vi "Main.vi"() -> ()   [LabVIEW 2014, in "TestFramework.lvlib"]
uses:
  TestFramework.lvlib
  FrontPanel/TypeDefs/clFrontPanelControlRefs.ctl
  WfrmGenerator/WfrmModule/WfrmModule.lvlib
  FGenModule/FGenModule.lvlib
  Bus/NISTBus.lvclass
  <userlib>/NIST/NISTErrorLib/NISTErrorLib.lvlib
  <vilib>/Utility/error.llb/Error Cluster From Error Code.vi
  <vilib>/ErrorRing/Error Ring.xnode
  FGenModule/PublicAPI/Arguments/Broadcasts/clErrorRpt.ctl
  WfrmGenerator/WfrmModule/PublicAPI/Arguments/Broadcasts/clErrorRpt.ctl
  WfrmGenerator/WfrmPlugins/EventPluginBaseClass/TypeDefs/dblEvtSignalArray.ctl
  WfrmGenerator/WfrmPlugins/EventPluginBaseClass/BaseWfrmPlugin.lvclass
  FGenPlugins/MyPluginBaseClass/TypeDef/PluginParams.ctl
  FGenPlugins/MyPluginBaseClass/NISTFGenPluginsBase.lvclass
  WfrmGenerator/WfrmPlugins/EventPluginBaseClass/TypeDefs/clEvtConfig.ctl
  WfrmGenerator/WfrmModule/PublicAPI/Arguments/Requests/dblEvtParams.ctl
  FGenPlugins/MyPluginBaseClass/TypeDef/CreateArbWfrmParams.ctl
  FGenPlugins/MyPluginBaseClass/TypeDef/ConfigArbWfrmParams.ctl
  FGenPlugins/MyPluginBaseClass/TypeDef/TriggerParams.ctl
panel:
  in  "btnSetTrigger":bool caption="btnLoadPlugin"
  in  "TriggerParams":T1={"eTrigger"=0, "eEdge"=10280, "sSource"=""} {"eEdge" items=["Rising"=10280, "Falling"=10171]; "eTrigger" items=["None", "Digital", "Analog"]}
  in  "EndTime":dbl=1.0
  in  "StartTime":dbl
  in  "btnClearArbWfrm":bool
  in  "ClrArbWfrmParams":cluster{"iIndex":i32}
  in  "btnInitialize":bool
  in  "btnReset":bool
  in  "btnSetOutputEnable":bool caption="btnLoadPlugin"
  in  "OutputEnableParams":cluster{"sName":string, "bEnabled":bool}
  in  "ConfigArbWfrmParams":T2={"sName"="1", "dGain"=2.0, "sWfrmHandle"="ARB1", "dOffset"=-1.0, "dSampleRate"=10000.0}
  in  "btnConfigWaveform":bool caption="btnLoadPlugin"
  in  "CreateArbWfrmParams":T3={"sName"="1", "iSize"=10000, "dData"=[], "sWfrmHandle"="ARB1"}
  in  "btnSendWaveform":bool caption="btnLoadPlugin"
  out "dblEventSignalArray":T4
  in  "dblEvtParams":T5=[[70.0, 70.0, 70.0, 70.0, 20.0, 20.0, 20.0, 20.0], [50.0, 60.0, 60.0, 60.0, 60.0, 60.0, 60.0, 60.0], [0.0, 0.0, 0.0, 0.0, 0.0, 0.0, 0.0, 0.0], [0.0, 0.0, 0.0, 0.0, 0.0, 0.0, 0.0, 0.0], [0.0, 0.0, 0.0, 0.0, 0.0, 0.0, 0.0, 0.0], [0.0, 0.0, 0.0, 0.0, 0.0, 0.0, 0.0, 0.0], [0.0, 0.0, 0.0, 0.0, 0.0, 0.0, 0.0, 0.0], [0.0, 0.0, 0.0, 0.0, 0.0, 0.0, 0.0, 0.0], [0.0, 0.0, 0.0, 0.0, 0.0, 0.0, 0.0, 0.0], [0.0, 0.0, 0.0, 0.0, 0.0, 0.0, 0.0, 0.0], [0.0, 0.0, 0.0, 0.0, 0.0, 0.0, 0.0, 0.0], [0.0, 0.0, 0.0, 0.0, 0.0, 0.0, 0.0, 0.0], [0.0, 0.0, 0.0, 0.0, 0.0, 0.0, 0.0, 0.0]]
  in  "clEvtConfig":T6={"T0(UTC)"=0.0, "F0"=60.0, "Fs"=60, "FSamp"=10000}
  in  "btnCreateWaveform":bool caption="btnLoadPlugin"
  in  "btnLoadWaveformPlugin":bool caption="btnLoadPlugin"
  in  "btnLoadPlugin":bool
  in  "Path to INI Waveform Plugin":path=path "../../EventPlugins/C37EvtPlugin/C37EvtPlugin.ini"
  in  "PluginParams":T7={"Path to Plugin INI"=path "../../MyPlugins/NiPxi6733/NiPxi6733.ini"}
  in  "btnRemoveBus":bool
  in  "btnSingleRun":bool
  out "Number of Buses":u8
  in  "Bus Number":u8(ring)
  in  "btnExit":bool
  in  "btnAddBus":bool
  # "Xm\nFin\nPs\nFh\nPh\nKh\nFa\nKa\nFx\nKx\nRf\nKaS\nKxS"
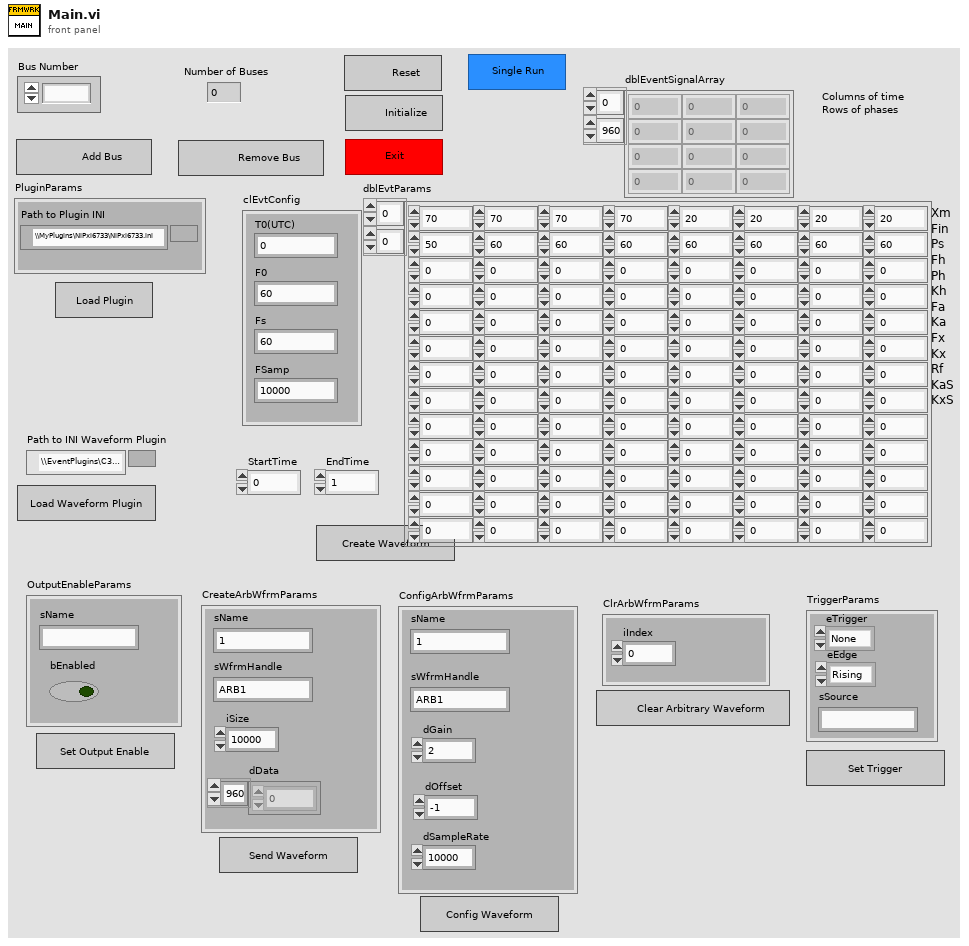
[diagram p1: front panel]
types:
  T1 = typedef "FGenPlugins.lvlib/NISTFGenPluginsBase.lvclass/TriggerParams.ctl" = cluster{"eTrigger":u16, "eEdge":u16, "sSource":string}
  T2 = typedef "FGenPlugins.lvlib/NISTFGenPluginsBase.lvclass/ConfigArbWfrmParams.ctl" = cluster{"sName":string, "dGain":dbl, "sWfrmHandle":string, "dOffset":dbl, "dSampleRate":dbl}
  T3 = typedef "FGenPlugins.lvlib/NISTFGenPluginsBase.lvclass/CreateArbWfrmParams.ctl" = cluster{"sName":string, "iSize":i32, "dData":dbl[], "sWfrmHandle":string}
  T4 = typedef "WfrmPlugins.lvlib/BaseWfrmPlugin.lvclass/dblEvtSignalArray.ctl" = dbl[][]
  T5 = typedef "WfrmModule.lvlib/dblEvtParams.ctl" = dbl[][]
  T6 = typedef "WfrmPlugins.lvlib/BaseWfrmPlugin.lvclass/clEvtConfig.ctl" = cluster{"T0(UTC)":dbl, "F0":dbl, "Fs":i32, "FSamp":u32}
  T7 = typedef "FGenPlugins.lvlib/NISTFGenPluginsBase.lvclass/PluginParams.ctl" = cluster{"Path to Plugin INI":path}
  T8 = typedef "TestFramework.lvlib/clFrontPanelControlRefs.ctl" = cluster{"BusNumberRef":refnum<vi>, "NumberOfBusesRef":refnum<vi>, "FGenPluginParamsRef":refnum<vi>, "WfrmINIFilePath":refnum<vi>, "EventSignalArrayRef":refnum<vi>, "CreateArbWfrmRef":refnum<vi>, "clEvtConFigRef":refnum<vi>, "dblEvtParamsRef":refnum<vi>, "clOutputEnableParamsRef":refnum<vi>, "ConfigArbWfrmRef":refnum<vi>, "ClArbWfrmParamsRef":refnum<vi>, "dStartTimeRef":refnum<vi>, "dEndTimeRef":refnum<vi>, "TriggerParamsRef":refnum<vi>}
  T9 = typedef "FGenModule.lvlib/clBroadcastEvents.ctl" = cluster{"DidInit":refnum<user-event>, "StatusUpdate":refnum<user-event>, "ErrorReport":refnum<user-event>, "DidStop":refnum<user-event>, "PathToINI":refnum<user-event>, "ChannelName":refnum<user-event>}
  T10 = typedef "WfrmModule.lvlib/clBroadcastEvents.ctl" = cluster{"DidInit":refnum<user-event>, "StatusUpdate":refnum<user-event>, "ErrorReport":refnum<user-event>, "DidStop":refnum<user-event>, "ReadEvtConfig":refnum<user-event>, "ReadTimeArray":refnum<user-event>, "ReadEvtParams":refnum<user-event>, "GetEvtReportArray":refnum<user-event>, "ReadPathToPlugin":refnum<user-event>, "GetEvtSignal":refnum<user-event>, "SendArbWfrm":refnum<user-event>}
  T11 = typedef "TestFramework.lvlib/clRequestEvents.ctl" = cluster{"StopRequest":refnum<user-event>}
  T12 = typedef "FGenModule.lvlib/clErrorRpt.ctl" = cluster{"error":errorcluster, "AdditionalInfo":string}
  T13 = typedef "WfrmModule.lvlib/clErrorRpt.ctl" = cluster{"error":errorcluster, "AdditionalInfo":string}
  T14 = typedef "TestFramework.lvlib/QueRef.ctl" = refnum<queue>
  T15 = typedef "TestFramework.lvlib/clFrameworkData.ctl" = cluster{"NISTBusClassInstances":refnum<class "NISTBus.lvclass">[], "NISTFGenINIFilePaths":path[], "NISTWfrmINIFilePaths":path[]}
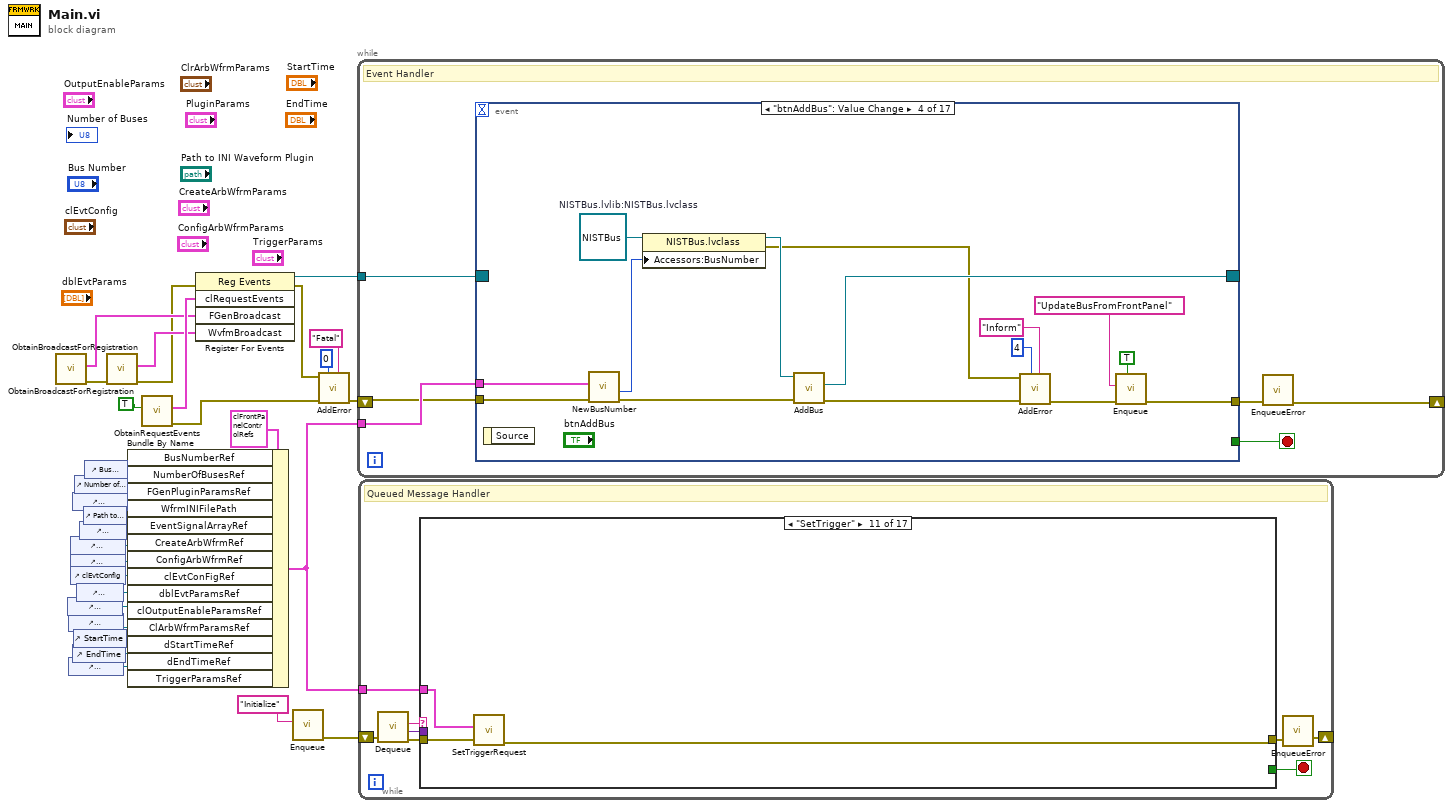
[diagram p0: block diagram]
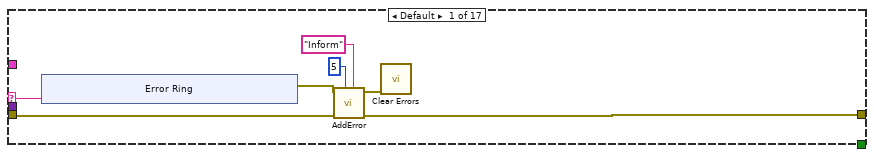
[diagram p2: hidden frame]
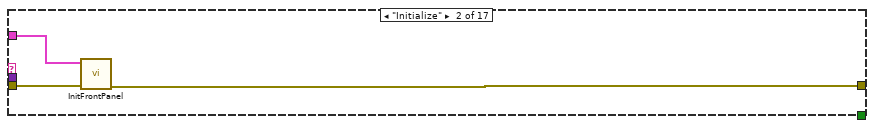
[diagram p3: hidden frame]
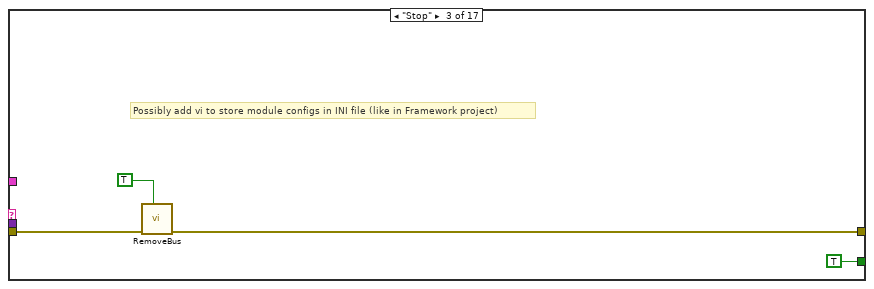
[diagram p4: hidden frame]
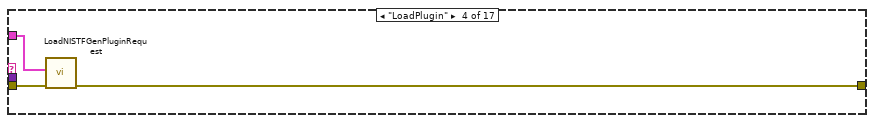
[diagram p5: hidden frame]
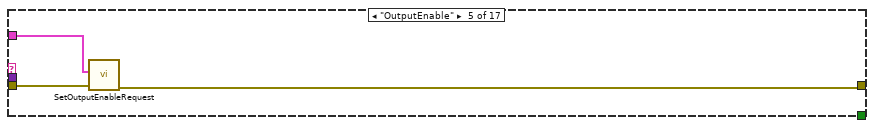
[diagram p6: hidden frame]
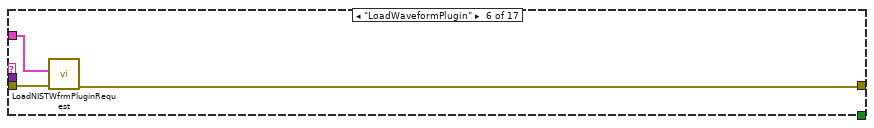
[diagram p7: hidden frame]
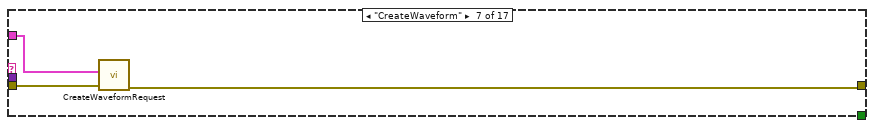
[diagram p8: hidden frame]
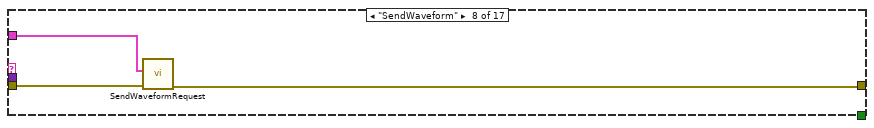
[diagram p9: hidden frame]
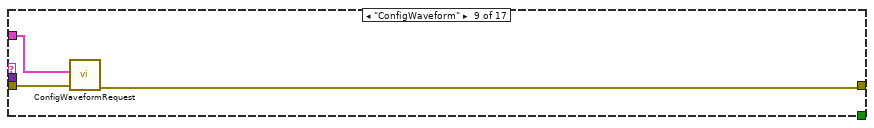
[diagram p10: hidden frame]
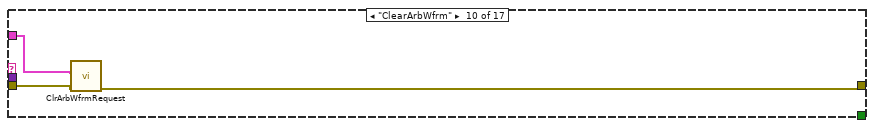
[diagram p11: hidden frame]
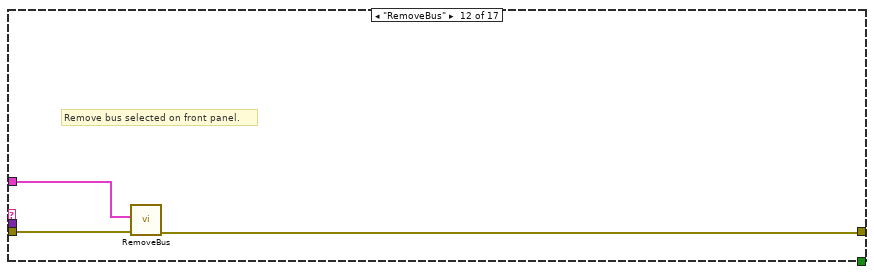
[diagram p12: hidden frame]
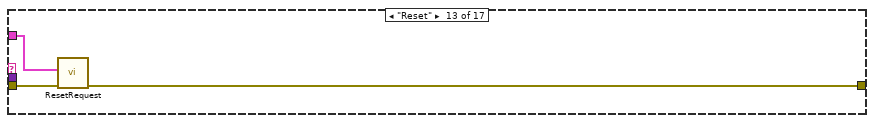
[diagram p13: hidden frame]
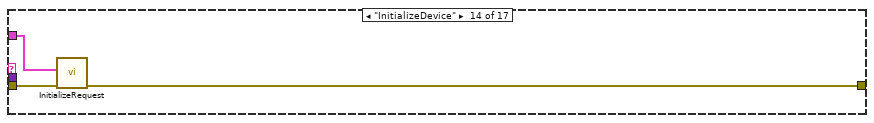
[diagram p14: hidden frame]
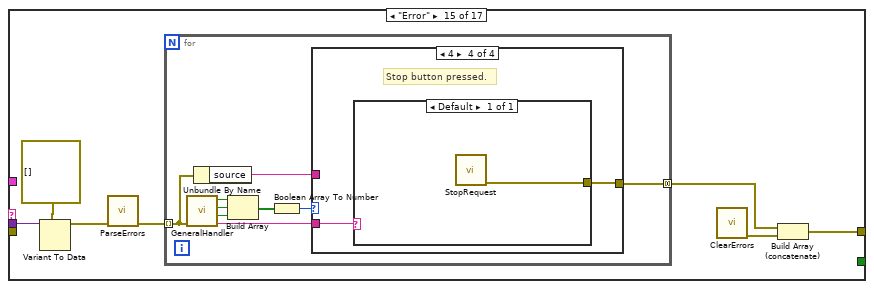
[diagram p15: hidden frame]
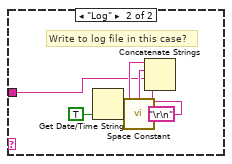
[diagram p18: hidden frame]
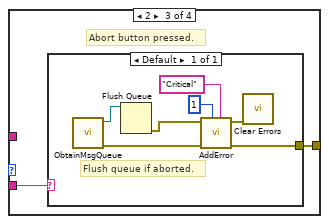
[diagram p19: hidden frame]
diagram:
  n1 = call "ObtainBroadcastForRegistration.vi"() -> ("error out"=w25:errorcluster, "FGenBroadcast"=w23:T9)  [unwired: 10 in]
  n2 = control-ref of="OutputEnableParams"() -> (w6:refnum<vi>)
  n3 = control-ref of="ClrArbWfrmParams"() -> (w4:refnum<vi>)
  n4 = control-ref of="TriggerParams"() -> (w1:refnum<vi>)
  n5 = control-ref of="CreateArbWfrmParams"() -> (w9:refnum<vi>)
  n6 = control-ref of="ConfigArbWfrmParams"() -> (w5:refnum<vi>)
  n7 = control-ref of="clEvtConfig"() -> (w8:refnum<vi>)
  n8 = control-ref of="PluginParams"() -> (w12:refnum<vi>)
  n9 = control-ref of="EndTime"() -> (w2:refnum<vi>)
  n10 = control-ref of="StartTime"() -> (w3:refnum<vi>)
  n11 = control-ref of="Number of Buses"() -> (w28:refnum<vi>)
  n12 = control-ref of="dblEvtParams"() -> (w7:refnum<vi>)
  n13 = control-ref of="dblEventSignalArray"() -> (w10:refnum<vi>)
  n14 = control-ref of="Path to INI Waveform Plugin"() -> (w11:refnum<vi>)
  n15 = control-ref of="Bus Number"() -> (w29:refnum<vi>)
  n16 = call "ObtainBroadcastForRegistration.vi"("error in (no error)"=w25) -> ("error out"=w22:errorcluster, "WvfmBroadcast"=w24:T10)  [unwired: 9 in]
  n17 = Bundle By Name(cluster=T8 {"BusNumberRef"=refnum, "NumberOfBusesRef"=refnum, "FGenPluginParamsRef"=refnum, "WfrmINIFilePath"=refnum, "EventSignalArrayRef"=refnum, "CreateArbWfrmRef"=refnum, "clEvtConFigRef"=refnum, "dblEvtParamsRef"=refnum, "clOutputEnableParamsRef"=refnum, "ConfigArbWfrmRef"=refnum, "ClArbWfrmParamsRef"=refnum, "dStartTimeRef"=refnum, "dEndTimeRef"=refnum, "TriggerParamsRef"=refnum} ("clFrontPanelControlRefs"), "BusNumberRef"=w29, "NumberOfBusesRef"=w28, "FGenPluginParamsRef"=w12, "WfrmINIFilePath"=w11, "EventSignalArrayRef"=w10, "CreateArbWfrmRef"=w9, "ConfigArbWfrmRef"=w5, "clEvtConFigRef"=w8, "dblEvtParamsRef"=w7, "clOutputEnableParamsRef"=w6, "ClArbWfrmParamsRef"=w4, "dStartTimeRef"=w3, "dEndTimeRef"=w2, "TriggerParamsRef"=w1) -> (w13:T8)
  n18 = call "ObtainRequestEvents.vi"("CreateNew (F)"=TRUE) -> ("ErrorArray Out"=w16:errorcluster[], "clRequestEvents"=w26:T11)  [unwired: 9 in]
  n19 = register-events(error in=w22, w26, w23, w24) -> (reference out=w21:refnum<event-registration>, error out=w17:errorcluster)  [unwired: 1 in]
  n20 = call "Enqueue.vi"("Msg"="Initialize") -> ("ErrorArray Out"=w14:errorcluster[])  [unwired: 10 in]
  n21 = call <userlib>:"AddError.vi"("Severity"="Fatal" ("String"), "Priority"=u8 0, "ErrorArray"=w16, "error in (no error)"=w17) -> ("ErrorArray"=w18:errorcluster[])  [unwired: 6 in, 1 out]
  n22 = while {
    tunnel: w21 -> [w35]
    tunnel: w13 -> [w34]
    shift-right: [w31] -> _
    shift-left: w18 -> [w33]
    stop <- w36 stop-if-true
    # "Event Handler"
    n23 = event shown="[3] \"btnAddBus\": Value Change" {
      selector: w35 -> [_ _ _ _ _ _ _ _ _ _ _ _ _ _ _ _ _]
      dyn-events: [_ _ _ w70 _ _ _ _ _ _ _ _ _ _ _ _ _] -> _
      timeout: _ -> [_ _ _ _ _ _ _ _ _ _ _ _ _ _ _ _ _]
      tunnel: [TRUE _ _ _ _ _ _ _ _ _ _ _ _ _ _ _ _] -> w36
      tunnel: w34 -> [_ _ _ w76 _ _ _ _ _ _ _ _ _ _ _ _ _]
      tunnel: w33 -> [w42 w45 w55 w73 w80 w83 w86 w89 w92 w95 w98 w101 w103 w106 w109 w113 w118]
      tunnel: [w39 w44 w54 w64 w79 w82 w85 w88 w91 w94 w97 w100 w102 w105 w108 w112 w117] -> w32
      event "btnExit": Value Change {
        n24 = event-data() -> ()  [unwired: 1 in, 1 out]
        n25 = call "RemoveBus.vi"("Remove All? (F)"=TRUE, "ErrorArray In"=w42) -> ("ErrorArray Out"=w40:errorcluster[])  [unwired: 9 in]
        n26 = call "Enqueue.vi"("Priority (f)"=TRUE, "ErrorArray In"=w40, "Msg"="Stop") -> ("ErrorArray Out"=w39:errorcluster[])  [unwired: 8 in]
      }
      event User Event {
        n27 = event-data() -> ("Data"=w46:variant)  [unwired: 1 in]
        n28 = Variant To Data(type=T12 {"error"={"status"=FALSE, "code"=0, "source"=""}, "AdditionalInfo"=""} ("Cluster"), Variant=w46) -> (data=w52:T12)  [unwired: 1 in, 1 out]
        n29 = Unbundle By Name(w52) -> ("error"=w48:errorcluster)
        n30 = call <userlib>:"AddError.vi"("Severity"="UserOption" ("String"), "Priority"=u8 2, "ErrorArray"=w45, "error in (no error)"=w48) -> ("ErrorArray"=w44:errorcluster[], "error out"=w49:errorcluster)  [unwired: 6 in]
        n31 = call <vilib>:"Clear Errors.vi"("error in (no error)"=w49) -> ()  [unwired: 5 in, 2 out]
      }
      event User Event {
        n32 = event-data() -> ("Data"=w61:variant)  [unwired: 1 in]
        n33 = Variant To Data(type=T13 {"error"={"status"=FALSE, "code"=0, "source"=""}, "AdditionalInfo"=""} ("Cluster"), Variant=w61) -> (data=w59:T13)  [unwired: 1 in, 1 out]
        n34 = Unbundle By Name(w59) -> ("error"=w53:errorcluster)
        n35 = call <userlib>:"AddError.vi"("Severity"="UserOption" ("String"), "Priority"=u8 2, "ErrorArray"=w55, "error in (no error)"=w53) -> ("ErrorArray"=w54:errorcluster[], "error out"=w56:errorcluster)  [unwired: 6 in]
        n36 = call <vilib>:"Clear Errors.vi"("error in (no error)"=w56) -> ()  [unwired: 5 in, 2 out]
      }
      event "btnAddBus": Value Change {
        w75 = refnum<class "NISTBus.lvclass"> refnum  # NISTBus.lvlib:NISTBus.lvclass
        n37 = event-data() -> ()  [unwired: 1 in, 1 out]
        n38 = call "NewBusNumber.vi"("ErrorArray In"=w73, "clFrontPanelControlRefs In"=w76) -> ("ErrorArray Out"=w71:errorcluster[], "BusNumber"=w74:u8)  [unwired: 7 in, 1 out]
        n39 = property class="NISTBus.lvclass"(reference=w75, "Accessors:BusNumber"=w74) -> (reference out=w72:refnum<class "NISTBus.lvclass">, error out=w67:errorcluster)  [unwired: 1 in]
        n40 = call "AddBus.vi"("ErrorArray In"=w71, "NISTBusClass In"=w72) -> ("ErrorArray Out"=w66:errorcluster[], "EvtReg"=w70:refnum<event-registration>)  [unwired: 7 in, 1 out]
        n41 = call <userlib>:"AddError.vi"("Severity"="Inform" ("String"), "Priority"=u8 4, "ErrorArray"=w66, "error in (no error)"=w67) -> ("ErrorArray"=w65:errorcluster[])  [unwired: 6 in, 1 out]
        n42 = call "Enqueue.vi"("Priority (f)"=TRUE, "ErrorArray In"=w65, "Msg"="UpdateBusFromFrontPanel") -> ("ErrorArray Out"=w64:errorcluster[])  [unwired: 8 in]
      }
      event "btnRemoveBus": Value Change {
        n43 = event-data() -> ()  [unwired: 1 in, 1 out]
        n44 = call "Enqueue.vi"("Priority (f)"=TRUE, "ErrorArray In"=w80, "Msg"="RemoveBus") -> ("ErrorArray Out"=w79:errorcluster[])  [unwired: 8 in]
      }
      event "btnReset": Value Change {
        n45 = event-data() -> ()  [unwired: 1 in, 1 out]
        n46 = call "Enqueue.vi"("ErrorArray In"=w83, "Msg"="Reset") -> ("ErrorArray Out"=w82:errorcluster[])  [unwired: 9 in]
      }
      event "btnInitialize": Value Change {
        n47 = event-data() -> ()  [unwired: 1 in, 1 out]
        n48 = call "Enqueue.vi"("ErrorArray In"=w86, "Msg"="InitializeDevice") -> ("ErrorArray Out"=w85:errorcluster[])  [unwired: 9 in]
      }
      event "btnSingleRun": Value Change {
        n49 = event-data() -> ()  [unwired: 1 in, 1 out]
        n50 = call "Enqueue.vi"("ErrorArray In"=w89, "Msg"="SingleRun") -> ("ErrorArray Out"=w88:errorcluster[])  [unwired: 9 in]
      }
      event "btnLoadPlugin": Value Change {
        n51 = event-data() -> ()  [unwired: 1 in, 1 out]
        n52 = call "Enqueue.vi"("ErrorArray In"=w92, "Msg"="LoadPlugin") -> ("ErrorArray Out"=w91:errorcluster[])  [unwired: 9 in]
      }
      event "btnSetOutputEnable": Value Change {
        n53 = event-data() -> ()  [unwired: 1 in, 1 out]
        n54 = call "Enqueue.vi"("ErrorArray In"=w95, "Msg"="OutputEnable") -> ("ErrorArray Out"=w94:errorcluster[])  [unwired: 9 in]
      }
      event "btnLoadWaveformPlugin": Value Change {
        n55 = event-data() -> ()  [unwired: 1 in, 1 out]
        n56 = call "Enqueue.vi"("ErrorArray In"=w98, "Msg"="LoadWaveformPlugin") -> ("ErrorArray Out"=w97:errorcluster[])  [unwired: 9 in]
      }
      event "btnCreateWaveform": Value Change {
        n57 = event-data() -> ()  [unwired: 1 in, 1 out]
        n58 = call "Enqueue.vi"("ErrorArray In"=w101, "Msg"="CreateWaveform") -> ("ErrorArray Out"=w100:errorcluster[])  [unwired: 9 in]
      }
      event "btnSendWaveform": Value Change {
        n59 = event-data() -> ()  [unwired: 1 in, 1 out]
        n60 = call "Enqueue.vi"("ErrorArray In"=w103, "Msg"="SendWaveform") -> ("ErrorArray Out"=w102:errorcluster[])  [unwired: 9 in]
      }
      event "btnConfigWaveform": Value Change {
        n61 = event-data() -> ()  [unwired: 1 in, 1 out]
        n62 = call "Enqueue.vi"("ErrorArray In"=w106, "Msg"="ConfigWaveform") -> ("ErrorArray Out"=w105:errorcluster[])  [unwired: 9 in]
      }
      event "btnClearArbWfrm": Value Change {
        n63 = event-data() -> ()  [unwired: 1 in, 1 out]
        n64 = call "Enqueue.vi"("ErrorArray In"=w109, "Msg"="ClearArbWfrm") -> ("ErrorArray Out"=w108:errorcluster[])  [unwired: 9 in]
      }
      event "btnSetTrigger": Value Change {
        n65 = event-data() -> ()  [unwired: 1 in, 1 out]
        n66 = call "Enqueue.vi"("ErrorArray In"=w113, "Msg"="SetTrigger") -> ("ErrorArray Out"=w112:errorcluster[])  [unwired: 9 in]
      }
      event User Event {
        n67 = event-data() -> ("Data"=w121:variant)  [unwired: 1 in]
        n68 = Variant To Data(type=T4 [] ("dblEventSignalArray"), Variant=w121) -> (data=→"dblEventSignalArray":T4, error out=w116:errorcluster)  [unwired: 1 in]
        n69 = call <userlib>:"AddError.vi"("Severity"="Inform" ("String"), "Priority"=u8 4, "ErrorArray"=w118, "error in (no error)"=w116) -> ("ErrorArray"=w117:errorcluster[])  [unwired: 6 in, 1 out]
      }
    }
    n70 = call "EnqueueError.vi"("ErrorArray In"=w32) -> ("ErrorArray Out"=w31:errorcluster[])  [unwired: 10 in]
  }
  n71 = while {
    shift-right: [w124] -> _
    shift-left: w14 -> [w128]
    tunnel: w13 -> [w129]
    stop <- w122 stop-if-true
    # "Queued Message Handler"
    n72 = call "Dequeue.vi"("ErrorArray In"=w128) -> ("ErrorArray Out"=w125:errorcluster[], "Data"=w126:variant, "Msg"=w127:string)  [unwired: 8 in]
    n73 = case shown="\"SetTrigger\"" w127 {
      selector: w127 -> [w130 _ _ _ _ _ _ _ _ _ _ _ _ _ _ _ _]
      tunnel: w129 -> [_ w146 _ w151 w154 w157 w160 w163 w166 w170 w173 w176 w180 w181 _ _ _]
      tunnel: w126 -> [_ _ _ _ _ _ _ _ _ _ _ _ _ _ w190 _ _]
      tunnel: w125 -> [w132 w145 w150 w153 w156 w159 w162 w165 w168 w169 w174 w177 w179 w182 _ w219 _]
      tunnel: [w131 w144 w149 w152 w155 w158 w161 w164 w167 w171 w172 w175 w178 w183 w185 w219 w220] -> w123
      tunnel: [_ _ TRUE _ _ _ _ _ _ _ _ _ _ _ _ _ _] -> w122
      frame Default {
        n74 = xnode "Error Ring"("parameter 0"=w130) -> ("error out"=w136:errorcluster)
        n75 = call <userlib>:"AddError.vi"("Severity"="Inform" ("String"), "Priority"=u8 5, "ErrorArray"=w132, "error in (no error)"=w136) -> ("ErrorArray"=w131:errorcluster[], "error out"=w133:errorcluster)  [unwired: 6 in]
        n76 = call <vilib>:"Clear Errors.vi"("error in (no error)"=w133) -> ()  [unwired: 5 in, 2 out]
      }
      frame "Initialize" {
        n77 = call "InitFrontPanel.vi"("ErrorArray In"=w145, "clFrontPanelControlRefs"=w146) -> ("ErrorArray Out"=w144:errorcluster[])  [unwired: 9 in]
      }
      frame "Stop" {
        # "Possibly add vi to store module configs in INI file (like in Framework project)"
        n78 = call "RemoveBus.vi"("Remove All? (F)"=TRUE, "ErrorArray In"=w150) -> ("ErrorArray Out"=w149:errorcluster[])  [unwired: 9 in]
      }
      frame "LoadPlugin" {
        n79 = call "LoadNISTFGenPluginRequest.vi"("ErrorArray In"=w153, "clFrontPanelControlRefs"=w151) -> ("ErrorArray Out"=w152:errorcluster[])  [unwired: 9 in]
      }
      frame "OutputEnable" {
        n80 = call "SetOutputEnableRequest.vi"("ErrorArray In"=w156, "clFrontPanelControlRefs"=w154) -> ("ErrorArray Out"=w155:errorcluster[])  [unwired: 9 in]
      }
      frame "LoadWaveformPlugin" {
        n81 = call "LoadNISTWfrmPluginRequest.vi"("ErrorArray In"=w159, "clFrontPanelControlRefs"=w157) -> ("ErrorArray Out"=w158:errorcluster[])  [unwired: 9 in]
      }
      frame "CreateWaveform" {
        n82 = call "CreateWaveformRequest.vi"("ErrorArray In"=w162, "clFrontPanelControlRefs"=w160) -> ("ErrorArray Out"=w161:errorcluster[])  [unwired: 9 in]
      }
      frame "SendWaveform" {
        n83 = call "SendWaveformRequest.vi"("ErrorArray In"=w165, "clFrontPanelControlRefs"=w163) -> ("ErrorArray Out"=w164:errorcluster[])  [unwired: 9 in]
      }
      frame "ConfigWaveform" {
        n84 = call "ConfigWaveformRequest.vi"("ErrorArray In"=w168, "clFrontPanelControlRefs"=w166) -> ("ErrorArray Out"=w167:errorcluster[])  [unwired: 9 in]
      }
      frame "ClearArbWfrm" {
        n85 = call "ClrArbWfrmRequest.vi"("ErrorArray In"=w169, "clFrontPanelControlRefs"=w170) -> ("ErrorArray Out"=w171:errorcluster[])  [unwired: 9 in]
      }
      frame "SetTrigger" {
        n86 = call "SetTriggerRequest.vi"("ErrorArray In"=w174, "clFrontPanelControlRefs"=w173) -> ("ErrorArray Out"=w172:errorcluster[])  [unwired: 9 in]
      }
      frame "RemoveBus" {
        # "Remove bus selected on front panel."
        n87 = call "RemoveBus.vi"("ErrorArray In"=w177, "clFrontPanelControlRefs"=w176) -> ("ErrorArray Out"=w175:errorcluster[])  [unwired: 9 in]
      }
      frame "Reset" {
        n88 = call "ResetRequest.vi"("ErrorArray In"=w179, "clFrontPanelControlRefs"=w180) -> ("ErrorArray Out"=w178:errorcluster[])  [unwired: 9 in]
      }
      frame "InitializeDevice" {
        n89 = call "InitializeRequest.vi"("ErrorArray In"=w182, "clFrontPanelControlRefs"=w181) -> ("ErrorArray Out"=w183:errorcluster[])  [unwired: 9 in]
      }
      frame "Error" {
        n90 = Variant To Data(type=errorcluster[] [], Variant=w190) -> (data=w188:errorcluster[])  [unwired: 1 in, 1 out]
        n91 = call <userlib>:"ParseErrors.vi"("ErrorArray"=w188) -> ("ErrorArray"=w187:errorcluster[])  [unwired: 8 in, 2 out]
        n92 = for {
          tunnel: w187 -> [w199] mode=indexing
          tunnel: [w191] -> w184 mode=concatenating
          n93 = call <userlib>:"GeneralHandler.vi"("error in (no error)"=w199) -> ("Severity"=w192:string, "Stop"=w196:bool, "Abort"=w197:bool, "Continue"=w198:bool)  [unwired: 7 in]
          n94 = Unbundle By Name(w199) -> ("source"=w193:string)
          n95 = Build Array(w198, w197, w196) -> (w194:bool[])
          n96 = Boolean Array To Number(Boolean array=w194) -> (number=w195:u32)
          n97 = case shown="4" w195 {
            tunnel: w193 -> [_ w200 _ _]
            tunnel: w192 -> [_ w201 w208 w217]
            tunnel: [_ _ w207 w216] -> w191
            frame 0, Default {
              # "No dialogue button pressed."
            }
            frame 1 {
              # "Continue button pressed."
              n98 = case shown="Default" w201 {
                tunnel: w200 -> [_ w202]
                frame Default {
                  # "Let the Framework continue."
                }
                frame "Log" {
                  # "Write to log file in this case?"
                  n99 = Get Date/Time String(want seconds? (F)=TRUE) -> (time string=w205:string)  [unwired: 2 in, 1 out]
                  n100 = call <vilib>:"Space Constant.vi"() -> ("String"=w204:string)
                  n101 = Concatenate Strings(w205, w204, w202, "\r\n") -> ()  [unwired: 1 out]
                }
              }
            }
            frame 2 {
              # "Abort button pressed."
              n102 = case shown="Default" w208 {
                tunnel: [w209] -> w207
                frame Default {
                  # "Flush queue if aborted."
                  n103 = call "ObtainMsgQueue.vi"() -> ("ErrorArray Out"=w211:errorcluster[], "QueRef"=w210:T14)  [unwired: 10 in]
                  n104 = Flush Queue(queue=w210) -> (error out=w215:errorcluster)  [unwired: 1 in, 2 out]
                  n105 = call <userlib>:"AddError.vi"("Severity"="Critical" ("String"), "Priority"=u8 1, "ErrorArray"=w211, "error in (no error)"=w215) -> ("ErrorArray"=w209:errorcluster[], "error out"=w212:errorcluster)  [unwired: 6 in]
                  n106 = call <vilib>:"Clear Errors.vi"("error in (no error)"=w212) -> ()  [unwired: 5 in, 2 out]
                }
              }
            }
            frame 4 {
              # "Stop button pressed."
              n107 = case shown="Default" w217 {
                tunnel: [w218] -> w216
                frame Default {
                  n108 = call "StopRequest.vi"() -> ("ErrorArray Out"=w218:errorcluster[])  [unwired: 11 in]
                }
              }
            }
          }
        }
        n109 = call <userlib>:"ClearErrors.vi"() -> ("ErrorArray"=w186:errorcluster[])  [unwired: 11 in]
        n110 = Build Array (concatenate)(w184, w186) -> (w185:errorcluster[])
      }
      frame "UpdateBusFromFrontPanel" {
        # "Incomplete (obviously)"
      }
      frame "SingleRun" {
        n111 = call "GetSetFrameworkData.vi"() -> ("clFrameworkData Out"=w222:T15)  [unwired: 11 in]
        n112 = Unbundle By Name(w222) -> ("NISTBusClassInstances"=w221:refnum<class "NISTBus.lvclass">[])
        n113 = for {
          tunnel: w221 -> [w227] mode=indexing
          tunnel: [w223] -> w220 mode=concatenating
          # "Incomplete"
          n114 = call "BuildRunScript.vi"("NISTBus In"=w227) -> ("ErrorArray Out"=w224:errorcluster[], "Script"=w225:string[], "NISTBus Out"=w226:refnum<class "NISTBus.lvclass">)  [unwired: 8 in]
          n115 = call "RunScript.vi"("ErrorArray In"=w224, "Script"=w225, "NISTBus In"=w226) -> ("ErrorArray Out"=w223:errorcluster[])  [unwired: 6 in, 2 out]
        }
      }
    }
    n116 = call "EnqueueError.vi"("ErrorArray In"=w123) -> ("ErrorArray Out"=w124:errorcluster[])  [unwired: 10 in]
  }
